vi "FRCts20_Backend_Event_PUT.vi"(6 "Message Attributes":T4, 8 "error in (no error)":errorcluster, 10 "Data":string, 11 "Engine_Refnums":T1) -> (0 "error out":errorcluster)   [LabVIEW 2013, in "FRCts20_Backend_Engine.lvlib"]
doc: "Updates the start time and end time of a specific event, called by the Event API. Expects an event index, start time, and end time"
uses:
  FRCts20_Backend_Engine.lvlib
  Dependencies/Keyed Array/KeyedArray.ctl
  FRCts20_Backend_EngineRefnums.ctl
  INI_Accessor/FRCts20_Backend_INI Controller.lvclass
  Dependencies/AMC/_SubVIs/TypeDefs/Message Queue.ctl
  Dependencies/AMC/_SubVIs/TypeDefs/Message.ctl
  <vilib>/addons/database/Connection.llb/Conn ObjectReference.ctl
  FRCts20_Backend_FGVOperation.ctl
  FRCts20_Backend_API/FRCts20_Backend_API_Event.ctl
  FRCts20_Backend_API/FRCts20_Backend_API_SW.ctl
  FRCts20_Backend_API/FRCts20_Backend_API.lvlib
  Dependencies/Keyed Array/Tools_KeyedArray.lvlib
  Dependencies/AMC/AMC.lvlib
  <vilib>/addons/database/NI_Database_API.lvlib
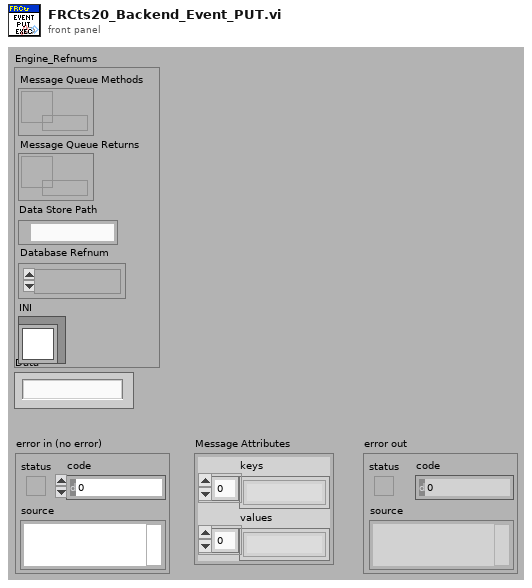
[diagram p1: front panel]
types:
  T1 = typedef "FRCts20_Backend_Engine.lvlib/FRCts20_Backend_EngineRefnums.ctl" = cluster{"Message Queue Methods":T2, "Message Queue Returns":T2, "Data Store Path":path, "Database Refnum":T3, "INI":refnum<class "FRCts20_Backend_INI Controller.lvclass">}
  T2 = typedef "AMC.lvlib/Message Queue.ctl" = refnum<queue>
  T3 = typedef "NI_Database_API.lvlib/Conn ObjectReference.ctl" = refnum<k1>
  T4 = typedef "Tools_KeyedArray.lvlib/KeyedArray.ctl" = cluster{"keys":string[], "values":string[]}
  T5 = typedef "FRCts20_Backend_API.lvlib/FRCts20_Backend_API_Event.ctl" = cluster{"Event Index":u32, "Name":string, "Start Time":timestamp, "End Time":timestamp, "Teams":cluster{"Team Index":u32, "Team Number":u32, "Requests":cluster{"Request Number":u32, "Description":string}[], "Has Open Issue":bool}[], "SWType":T6, "APIReturn":string}
  T6 = typedef "FRCts20_Backend_API.lvlib/FRCts20_Backend_API_SW.ctl" = string
  T7 = typedef "FRCts20_Backend_Engine.lvlib/FRCts20_Backend_FGVOperation.ctl" = enum16{"Initialize", "EnqueueMessage", "EnqueueDataReturn", "FlushMessage", "FlushDataReturn"}
  T8 = cluster{"Team Index":u32, "Team Number":u32, "Requests":cluster{"Request Number":u32, "Description":string}[], "Has Open Issue":bool}[]
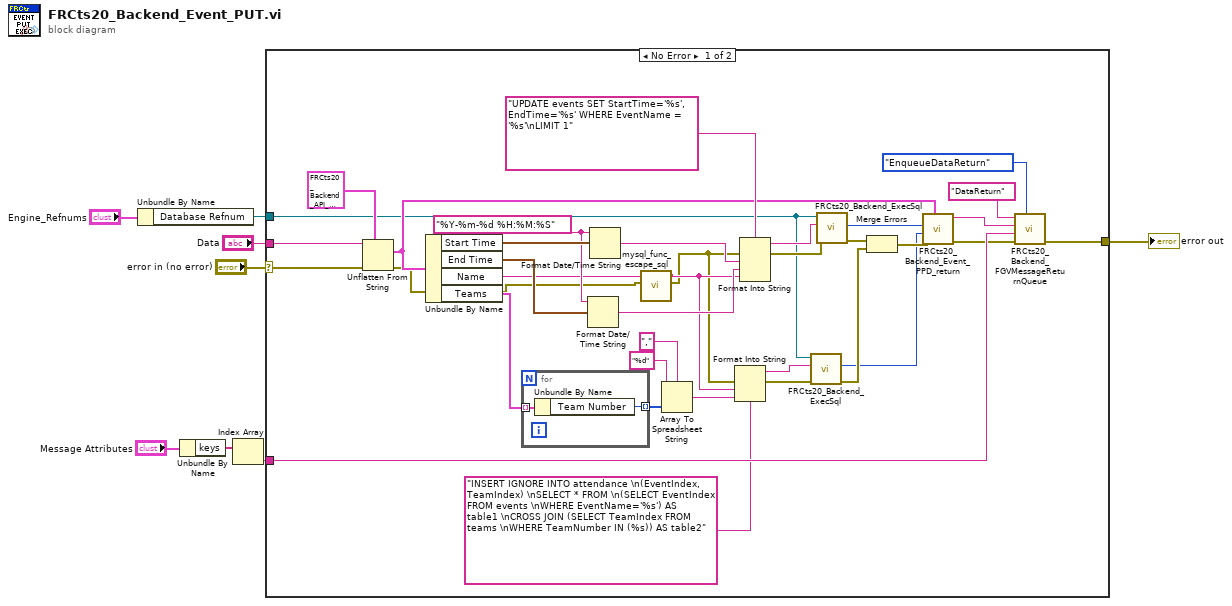
[diagram p0: block diagram]
diagram:
  n1 = Unbundle By Name("Engine_Refnums") -> ("Database Refnum"=w5:T3)
  n2 = Unbundle By Name("Message Attributes") -> ("keys"=w2:string[])
  n3 = Index Array(array=w2) -> (element=w1:string)  [unwired: 1 in]
  n4 = case shown="No Error" "error in (no error)" {
    selector: "error in (no error)" -> [w41 w47]
    tunnel: [w44 w47] -> w7
    tunnel: w5 -> [w20 _]
    tunnel: "Data" -> [w42 _]
    tunnel: w1 -> [w43 _]
    frame No Error {
      w14 = "%Y-%m-%d %H:%M:%S" ("time format string (%c)")
      n5 = Unflatten From String(type=T5 {"Event Index"=0, "Name"="", "Start Time"=timestamp(0 s since 1904-01-01), "End Time"=timestamp(0 s since 1904-01-01), "Teams"=[], "SWType"="", "APIReturn"=""} ("Competition"), binary string=w42, error in (no error)=w41) -> (value=w31:T5, error out=w10:errorcluster)  [unwired: 2 in, 1 out]
      n6 = Unbundle By Name(w31) -> ("Start Time"=w36:timestamp, "End Time"=w28:timestamp, "Name"=w12:string, "Teams"=w27:T8)
      n7 = for {
        tunnel: w27 -> [w46] mode=indexing
        tunnel: [w45] -> w26 mode=indexing
        n8 = Unbundle By Name(w46) -> ("Team Number"=w45:u32)
      }
      n9 = Format Date/Time String(time format string (%c)=w14, seconds (now)=w28) -> (date/time string=w22:string)  [unwired: 1 in]
      n10 = Format Date/Time String(time format string (%c)=w14, seconds (now)=w36) -> (date/time string=w35:string)  [unwired: 1 in]
      n11 = call "mysql_func_escape_sql.vi"("error in (no error)"=w10, "sqlin"=w12) -> ("error out"=w9:errorcluster, "escaped"=w11:string)  [unwired: 8 in]
      n12 = Array To Spreadsheet String(delimiter (Tab)=",", array=w26, 3:"%d" ("format string")) -> (spreadsheet string=w21:string)
      n13 = Format Into String(format string="INSERT IGNORE INTO attendance \n(EventIndex, TeamIndex) \nSELECT * FROM \n(SELECT EventIndex FROM events \nWHERE EventName='%s') AS table1 \nCROSS JOIN (SELECT TeamIndex FROM teams \nWHERE TeamNumber IN (%s)) AS table2", error in=w9, w11, w21) -> (resulting string=w19:string, error out=w18:errorcluster)  [unwired: 1 in]
      n14 = Format Into String(format string="UPDATE events SET StartTime='%s', EndTime='%s' WHERE EventName = '%s'\nLIMIT 1", error in=w9, w35, w22, w11) -> (resulting string=w33:string, error out=w32:errorcluster)  [unwired: 1 in]
      n15 = call "FRCts20_Backend_ExecSql.vi"("error in (no error)"=w18, "format string"=w19, "Refnum in"=w20) -> ("error out"=w16:errorcluster, "rows affected"=w13:i32)  [unwired: 6 in, 1 out]
      n16 = call "FRCts20_Backend_ExecSql.vi"("error in (no error)"=w32, "format string"=w33, "Refnum in"=w20) -> ("error out"=w17:errorcluster, "rows affected"=w34:i32)  [unwired: 6 in, 1 out]
      n17 = Merge Errors(w17, w16) -> (w15:errorcluster)
      n18 = call "FRCts20_Backend_Event_PPD_return.vi"("Event"=w31, "error in (no error)"=w15, "rows affected 2"=w13, "rows affected"=w34) -> ("error out"=w30:errorcluster, "data string"=w29:string)  [unwired: 6 in]
      n19 = call "FRCts20_Backend_FGVMessageReturnQueue.vi"("Operation"=FRCts20_Backend_FGVOperation."EnqueueDataReturn", "error in (no error)"=w30, "Key"=w43, "Message Value"=w29, "Message Name"="DataReturn") -> ("error out"=w44:errorcluster)  [unwired: 5 in, 1 out]
    }
    frame Error {
    }
  }
  "error out" <- w7
